vi "LVSWrt_Rd_Trm.vi"(9 "WriteBuf":string="?", 11 "COM Port":refnum<visa-resource-name>) -> (0 "ComError":bool, 2 "string read":string)   [LabVIEW 2013]
uses:
  instr.lib/lvserial/lvserial.lvlib
  <vilib>/Utility/error.llb/DialogType.ctl
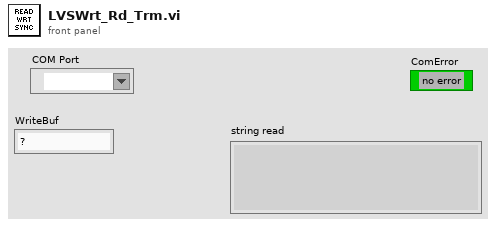
[diagram p1: front panel]
types:
  T1 = typedef "DialogType.ctl" = u16
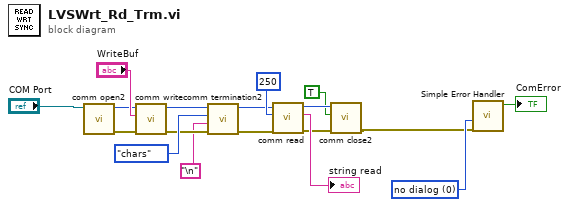
[diagram p0: block diagram]
diagram:
  w3 = T1 0 items=["no dialog", "OK message", "continue or stop message", "OK message + warnings", "continue/stop + warnings"] ("type of dialog (OK msg:1)")
  n1 = call "comm open2.vi"("Comm Port Name"="COM Port") -> ("error out"=w14:errorcluster, "Comm Handle"=w13:u32)  [unwired: 4 in, 1 out]
  n2 = call "comm write.vi"("error in (no error)"=w14, "string to write"="WriteBuf", "Comm Handle"=w13) -> ("error out"=w9:errorcluster, "dup Comm Handle"=w10:u32)  [unwired: 6 in, 1 out]
  n3 = call "comm termination2.vi"("error in (no error)"=w9, "termination"="\n", "Termination Mode"=enum16{"none", "chars", "string", "regex"}."chars", "Comm Handle"=w10) -> ("error out"=w6:errorcluster, "dup Comm Handle"=w7:u32)  [unwired: 6 in]
  n4 = call "comm read.vi"("error in (no error)"=w6, "requested byte count"=u32 250, "Comm Handle"=w7) -> ("error out"=w12:errorcluster, "string read"=→"string read":string, "dup Comm Handle"=w17:u32)  [unwired: 5 in, 1 out]
  n5 = call "comm close2.vi"("error in (no error)"=w12, "close all? (F)"=TRUE, "Comm Handle"=w17) -> ("error out"=w1:errorcluster)  [unwired: 4 in]
  n6 = call <vilib>:"Simple Error Handler.vi"("type of dialog (OK msg:1)"=w3, "error in (no error)"=w1) -> ("error?"=→"ComError":bool)  [unwired: 7 out]
